vi "Read Service Name.vi"(8 "error in (no error)":errorcluster, 11 "WebSocket Service in":refnum<class "WebSocket Service.lvclass">) -> (0 "error out":errorcluster, 2 "Service Name":string, 3 "WebSocket Service out":refnum<class "WebSocket Service.lvclass">)   [LabVIEW 2016, in "WebSocket Actors.lvlib" / "WebSocket Service.lvclass"]
uses:
  WebSocket Service.lvclass
  WebSocket Service.lvclass/WebSocket Service.ctl
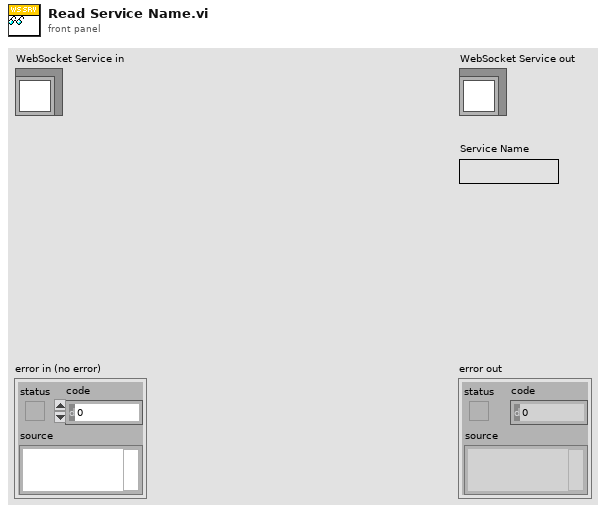
[diagram p1: front panel]
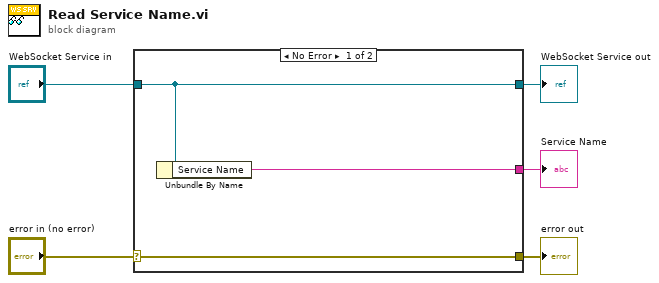
[diagram p0: block diagram]
diagram:
  n1 = case shown="No Error" "error in (no error)" {
    selector: "error in (no error)" -> [w8 w9]
    tunnel: [w8 w9] -> w4
    tunnel: [w7 w10] -> w2
    tunnel: "WebSocket Service in" -> [w7 w10]
    tunnel: [w6 _] -> w1
    frame No Error {
      n2 = Unbundle By Name(w7) -> ("Service Name"=w6:string)
    }
    frame Error {
    }
  }
  "error out" <- w4
  "WebSocket Service out" <- w2
  "Service Name" <- w1
